vi "CFTS-Store Acoustic System IDs.vi"(8 "error in (no error)":errorcluster, 10 "Left":string, 11 "Right":string) -> (0 "error out":errorcluster)   [LabVIEW 2020]
uses:
  <vilib>/Utility/config.llb/Write Key (String).vi
  <vilib>/Utility/config.llb/NI_LVConfig.lvlib
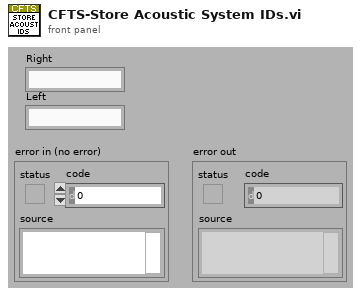
[diagram p1: front panel]
types:
  T1 = typedef "NI_LVConfig.lvlib/Config Data RefNum.ctl" = refnum<k1>
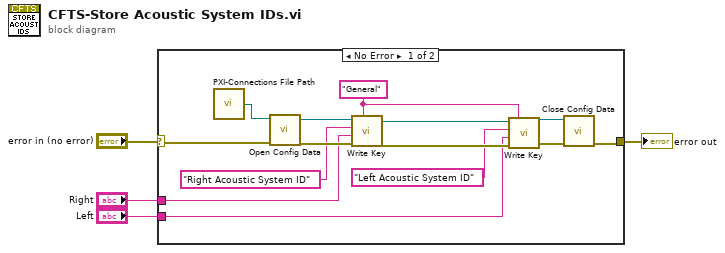
[diagram p0: block diagram]
diagram:
  n1 = case shown="No Error" "error in (no error)" {
    selector: "error in (no error)" -> [w18 w19]
    tunnel: [w10 w19] -> w4
    tunnel: "Right" -> [w7 _]
    tunnel: "Left" -> [w6 _]
    frame No Error {
      w14 = "General" ("section")
      n2 = call "PXI-Connections File Path.vi"() -> ("Path"=w5:path)  [unwired: 1 in]
      n3 = call <vilib>:"Open Config Data.vi"("error in (no error)"=w18, "configuration file path"=w5) -> ("error out"=w17:errorcluster, "refnum"=w16:T1)  [unwired: 7 in, 1 out]
      n4 = call-poly <vilib>:"Write Key.vi"("section"=w14, "error in (no error)"=w17, "value"=w7, "key"="Right Acoustic System ID", "refnum"=w16) -> ("error out"=w12:errorcluster, "refnum out"=w13:T1)  [unwired: 4 in, 1 out]
      n5 = call-poly <vilib>:"Write Key.vi"("section"=w14, "error in (no error)"=w12, "value"=w6, "key"="Left Acoustic System ID", "refnum"=w13) -> ("error out"=w9:errorcluster, "refnum out"=w8:T1)  [unwired: 4 in, 1 out]
      n6 = call <vilib>:"Close Config Data.vi"("error in (no error)"=w9, "refnum"=w8) -> ("error out"=w10:errorcluster)  [unwired: 8 in, 1 out]
    }
    frame Error {
    }
  }
  "error out" <- w4
